vi "AccelerometerSampleFIFOSync.vi"(0 "Output type":i16=1, 1 "Period (ms)":u32=5) -> (2 "Ticks":i32, 3 "FIFO full":bool, 4 "Timeouted":bool)   [LabVIEW 2018]
uses:
  <vilib>/rvi/Emulation/niFpgaGetClockAttributes.vi
  <vilib>/rvi/Emulation/niFpgaSctlEmulationGetInTimedLoop.vi
  <vilib>/rvi/Emulation/niFpgaEmulationReportErrorSimple.vi
  <vilib>/rvi/eio/common/nirviEmuTemplateMethod_errors.vi
  <vilib>/rvi/occurrence/nirviWaitOnOccurrenceBase.vi
  <vilib>/rvi/Emulation/niFpgaCriticalErrorInLSC.vi
  <vilib>/rvi/Emulation/niFpgaProcessEmulError.vi
  <vilib>/rvi/Emulation/niFpgaEmulationIsFPGAContextNoSignature.vi
  <vilib>/rvi/errors/niFpgaSetErrorForExecOnDevCompSimple.vi
  <vilib>/rvi/eio/common/nirviEmuReportErrorAndStop.vi
  <vilib>/rvi/DataTransferAndStorage/Container/Common/niFpgaContainerGetUniqueNameForEmu.vi
  <vilib>/rvi/FIFO/Fifo_Resource/nirvififoEmulationSetSize.vi
  <vilib>/rvi/FIFO/Fifo_Resource/nirviFifoEmulationQueueMgr.vi
  <instcachedir>/0/nirviFifoEmulationQueueMgr_E5CAEC123FF24DC58D834DCA3CDAA9B5.lvgen/nirviFifoEmulationQueueMgr_E5CAEC123FF24DC58D834DCA3CDAA9B5_005.vi
  <vilib>/Utility/error.llb/Clear Errors.vi
  <vilib>/rvi/FIFO/Fifo_Resource/nirvififoEmulationCreateLock.vi
  <vilib>/rvi/FIFO/Fifo_Resource/nirvififoEmulationObtainLock.vi
  <vilib>/rvi/FIFO/Fifo_Resource/nirvififoEmulationReleaseLock.vi
  <vilib>/rvi/errors/nirviReportUnexpectedCaseInternalError.vi
  <vilib>/rvi/errors/nirviReportUnexpectedCaseInternalError (U32).vi
  <vilib>/eio/EIONode/EIONode.xnode
  <vilib>/rvi/DataTransferAndStorage/Container/XNode/niFpgaContainer.xnode
  <vilib>/rvi/FIFO/Fifo_Resource/nirvififoEmulationRead.vi
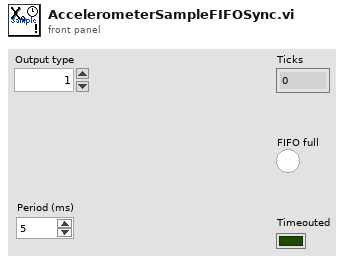
[diagram p1: front panel]
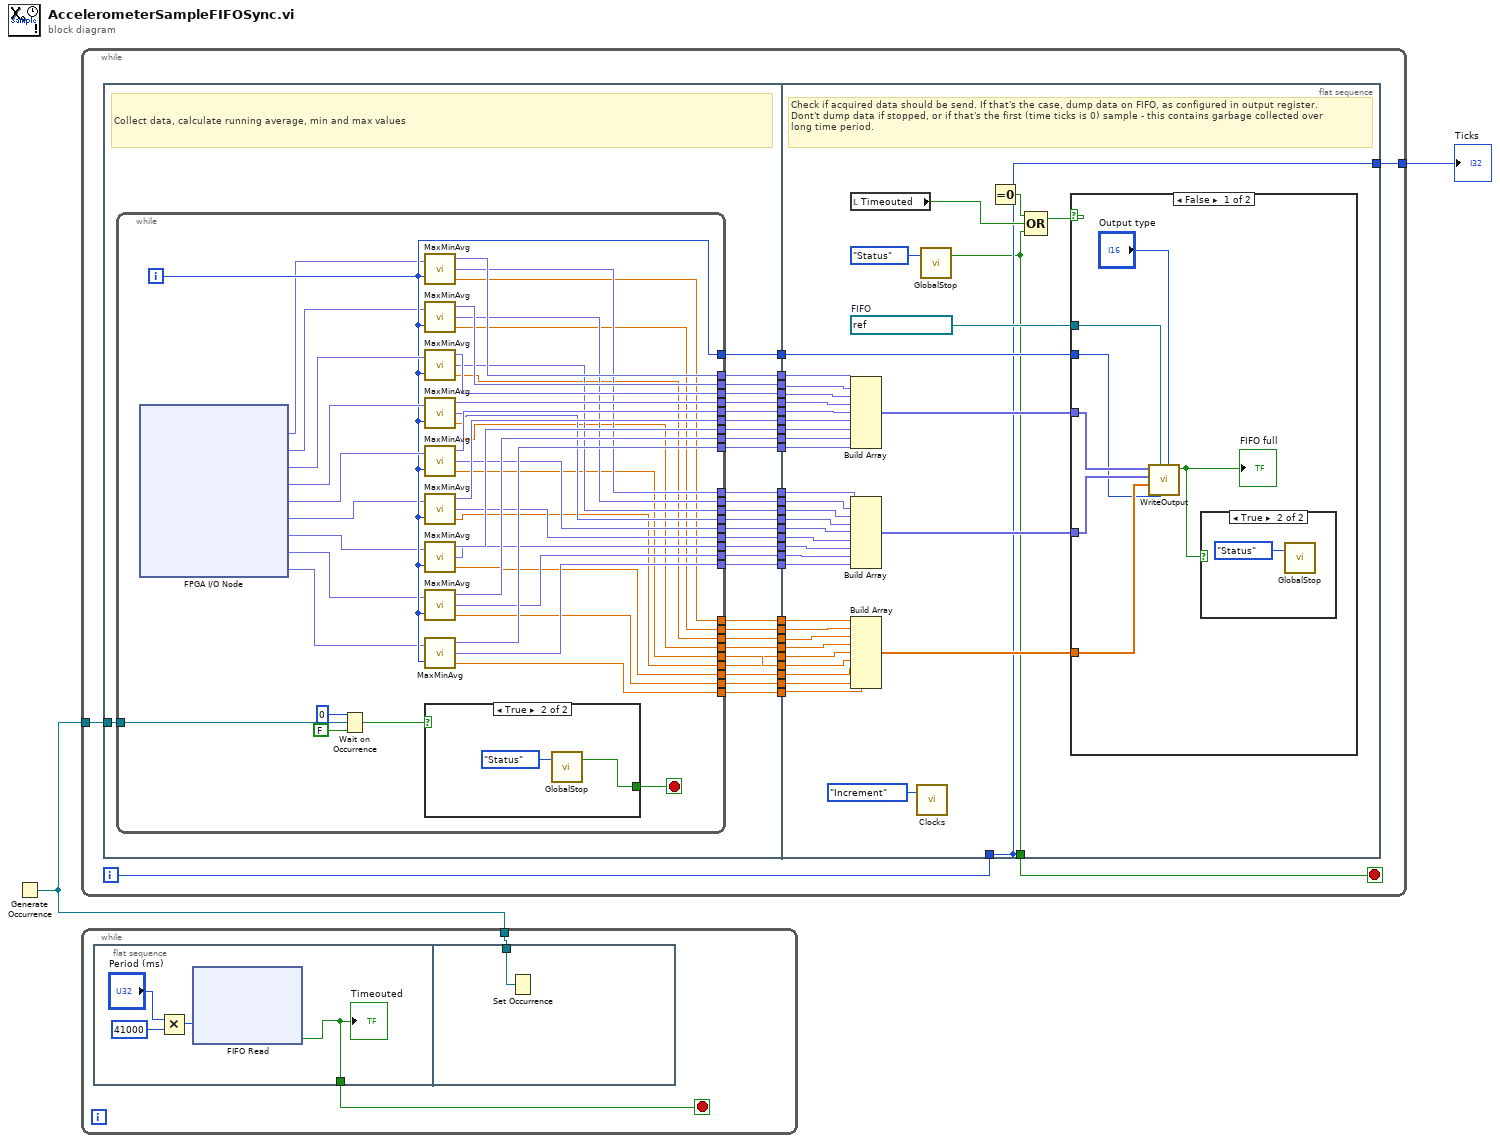
[diagram p0: block diagram]
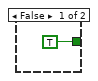
[diagram p2: hidden frame]
diagram:
  n1 = Generate Occurrence() -> (w2:refnum<k4>)
  n2 = while {
    tunnel: w2 -> [w5]
    tunnel: [w3] -> w1
    i -> [w4]
    stop <- w7 stop-if-true
    n3 = flat-sequence {
      tunnel: [w63] -> w34
      tunnel: [w62] -> w33
      tunnel: [w61] -> w32
      tunnel: [w60] -> w31
      tunnel: [w59] -> w30
      tunnel: [w58] -> w29
      tunnel: [w57] -> w28
      tunnel: [w56] -> w27
      tunnel: [w55] -> w26
      tunnel: [w54] -> w25
      tunnel: [w53] -> w24
      tunnel: [w52] -> w23
      tunnel: [w51] -> w22
      tunnel: [w50] -> w21
      tunnel: [w49] -> w20
      tunnel: [w48] -> w19
      tunnel: [w47] -> w18
      tunnel: [w46] -> w17
      tunnel: [w45] -> w16
      tunnel: [w44] -> w15
      tunnel: [w43] -> w14
      tunnel: [w42] -> w13
      tunnel: [w41] -> w12
      tunnel: [w40] -> w11
      tunnel: [w39] -> w10
      tunnel: [w38] -> w9
      tunnel: [w37] -> w8
      tunnel: [w36] -> w6
      tunnel: w5 -> [w35]
      tunnel: w34 -> [w147]
      tunnel: w33 -> [w146]
      tunnel: w32 -> [w145]
      tunnel: w31 -> [w144]
      tunnel: w30 -> [w143]
      tunnel: w29 -> [w142]
      tunnel: w28 -> [w141]
      tunnel: w27 -> [w140]
      tunnel: w26 -> [w139]
      tunnel: w25 -> [w138]
      tunnel: w24 -> [w137]
      tunnel: w23 -> [w136]
      tunnel: w22 -> [w135]
      tunnel: w21 -> [w134]
      tunnel: w20 -> [w133]
      tunnel: w19 -> [w132]
      tunnel: w18 -> [w131]
      tunnel: w17 -> [w130]
      tunnel: w16 -> [w129]
      tunnel: w15 -> [w128]
      tunnel: w14 -> [w127]
      tunnel: w13 -> [w126]
      tunnel: w12 -> [w121]
      tunnel: w11 -> [w122]
      tunnel: w10 -> [w125]
      tunnel: w9 -> [w124]
      tunnel: w8 -> [w123]
      tunnel: [w110] -> w7
      tunnel: w6 -> [w113]
      tunnel: w4 -> [w112]
      tunnel: [w112] -> _
      tunnel: [w112] -> w3
      frame #0 {
        # "Collect data, calculate running average, min and max values"
        n4 = while {
          tunnel: [w102] -> w63
          tunnel: [w101] -> w62
          tunnel: [w100] -> w61
          tunnel: [w99] -> w60
          tunnel: [w98] -> w59
          tunnel: [w97] -> w58
          tunnel: [w96] -> w57
          tunnel: [w95] -> w56
          tunnel: [w94] -> w55
          tunnel: [w93] -> w54
          tunnel: [w92] -> w53
          tunnel: [w91] -> w52
          tunnel: [w90] -> w51
          tunnel: [w89] -> w50
          tunnel: [w88] -> w49
          tunnel: [w87] -> w48
          tunnel: [w86] -> w47
          tunnel: [w85] -> w46
          tunnel: [w84] -> w45
          tunnel: [w83] -> w44
          tunnel: [w82] -> w43
          tunnel: [w81] -> w42
          tunnel: [w80] -> w41
          tunnel: [w79] -> w40
          tunnel: [w78] -> w39
          tunnel: [w77] -> w38
          tunnel: [w76] -> w37
          tunnel: [w75] -> w36
          tunnel: w35 -> [w72]
          i -> [w75]
          stop <- w74 stop-if-true
          n5 = xnode "FPGA I/O Node"() -> ("Accelerometer1/AI0"=w65:fxp<+/-,24,7>, "Accelerometer1/AI1"=w69:fxp<+/-,24,7>, "Accelerometer1/AI2"=w105:fxp<+/-,24,7>, "Accelerometer2/AI0"=w104:fxp<+/-,24,7>, "Accelerometer2/AI1"=w103:fxp<+/-,24,7>, "Accelerometer2/AI2"=w66:fxp<+/-,24,7>, "Accelerometer3/AI0"=w67:fxp<+/-,24,7>, "Accelerometer3/AI1"=w68:fxp<+/-,24,7>, "Accelerometer3/AI2"=w64:fxp<+/-,24,7>)  [unwired: 9 in, 9 out]
          n6 = Wait on Occurrence(1:FALSE ("ignore previous (T)"), 2:w72, 3:0 ("ms timeout (-1)")) -> (0:w73:bool)
          n7 = call "MaxMinAvg.vi"("Measurement"=w65, "Index"=w75) -> ("Minimum Value"=w102:fxp<+/-,24,4>, "Maximum Value"=w93:fxp<+/-,24,4>, "Average Value"=w84:sgl)
          n8 = call "MaxMinAvg.vi"("Measurement"=w69, "Index"=w75) -> ("Minimum Value"=w101:fxp<+/-,24,4>, "Maximum Value"=w92:fxp<+/-,24,4>, "Average Value"=w83:sgl)
          n9 = call "MaxMinAvg.vi"("Measurement"=w105, "Index"=w75) -> ("Minimum Value"=w100:fxp<+/-,24,4>, "Maximum Value"=w91:fxp<+/-,24,4>, "Average Value"=w82:sgl)
          n10 = call "MaxMinAvg.vi"("Measurement"=w104, "Index"=w75) -> ("Minimum Value"=w99:fxp<+/-,24,4>, "Maximum Value"=w90:fxp<+/-,24,4>, "Average Value"=w81:sgl)
          n11 = call "MaxMinAvg.vi"("Measurement"=w103, "Index"=w75) -> ("Minimum Value"=w98:fxp<+/-,24,4>, "Maximum Value"=w89:fxp<+/-,24,4>, "Average Value"=w80:sgl)
          n12 = call "MaxMinAvg.vi"("Measurement"=w66, "Index"=w75) -> ("Minimum Value"=w97:fxp<+/-,24,4>, "Maximum Value"=w88:fxp<+/-,24,4>, "Average Value"=w79:sgl)
          n13 = call "MaxMinAvg.vi"("Measurement"=w67, "Index"=w75) -> ("Minimum Value"=w96:fxp<+/-,24,4>, "Maximum Value"=w87:fxp<+/-,24,4>, "Average Value"=w78:sgl)
          n14 = call "MaxMinAvg.vi"("Measurement"=w68, "Index"=w75) -> ("Minimum Value"=w95:fxp<+/-,24,4>, "Maximum Value"=w86:fxp<+/-,24,4>, "Average Value"=w77:sgl)
          n15 = call "MaxMinAvg.vi"("Measurement"=w64, "Index"=w75) -> ("Minimum Value"=w94:fxp<+/-,24,4>, "Maximum Value"=w85:fxp<+/-,24,4>, "Average Value"=w76:sgl)
          n16 = case shown="True" w73 {
            tunnel: [TRUE w107] -> w74
            frame False {
            }
            frame True {
              n17 = call "GlobalStop.vi"("Enum"=enum16{"Clear", "Set", "Status"}."Status") -> ("Boolean"=w107:bool)  [unwired: 1 in, 1 out]
            }
          }
        }
      }
      frame #1 {
        w120 = refnum<k21> "ResponseFIFO"  # FIFO
        # "Check if acquired data should be send. If that's the case, dump data on FIFO, as configured in output register.\nDont't dump data if stopped, or if that's the first (time ticks is 0) sample - this contains garbage collected over\nlong time period."
        n18 = local read "Timeouted"() -> (w114:bool)
        n19 = Build Array(w147, w146, w145, w144, w143, w142, w141, w140, w139) -> (w119:fxp<+/-,24,4>[])
        n20 = Build Array(w138, w137, w136, w135, w134, w133, w132, w131, w130) -> (w118:fxp<+/-,24,4>[])
        n21 = Build Array(w129, w128, w127, w126, w122, w121, w125, w124, w123) -> (w117:sgl[])
        n22 = call "Clocks.vi"("Enum"=enum16{"Reset", "Increment", "Get"}."Increment") -> ()  [unwired: 1 in, 2 out]
        n23 = call "GlobalStop.vi"("Enum"=enum16{"Clear", "Set", "Status"}."Status") -> ("Boolean"=w110:bool)  [unwired: 1 in, 1 out]
        n24 = Equal To 0?(x=w112) -> (x = 0?=w115:bool)
        n25 = Compound Arithmetic op=OR(w115, w114, w110) -> (w116:bool)
        n26 = case shown="False" w116 {
          tunnel: w120 -> [w154 _]
          tunnel: w119 -> [w153 _]
          tunnel: w118 -> [w152 _]
          tunnel: w117 -> [w151 _]
          tunnel: w113 -> [w150 _]
          frame False {
            n27 = call "WriteOutput.vi"("Output type"="Output type", "Number of Samples"=w150, "Output FIFO"=w154, "Average"=w151, "Max"=w152, "Min"=w153) -> ("FIFO full"=w148:bool)  [unwired: 5 in]
            "FIFO full" <- w148
            n28 = case shown="True" w148 {
              frame False {
              }
              frame True {
                n29 = call "GlobalStop.vi"("Enum"=enum16{"Clear", "Set", "Status"}."Status") -> ()  [unwired: 1 in, 2 out]
              }
            }
          }
          frame True {
          }
        }
      }
    }
  }
  "Ticks" <- w1
  n30 = while {
    tunnel: w2 -> [w156]
    stop <- w157 stop-if-true
    n31 = flat-sequence {
      tunnel: [w161] -> w157
      tunnel: w156 -> [w162]
      frame #0 {
        n32 = Multiply(x="Period (ms)", y=u32 41000) -> (x*y=w160:u32)
        n33 = xnode "FIFO Read"("Timeout"=w160) -> ("Timed Out?"=w161:bool)  [unwired: 1 in, 2 out]
        "Timeouted" <- w161
      }
      frame #1 {
        n34 = Set Occurrence(w162) -> ()
      }
    }
  }
